vi "Close.vi"(8 "error in":errorcluster, 11 "Current Gradient in":refnum<class "Current Gradient.lvclass">) -> (0 "error out":errorcluster, 3 "Current Gradient out":refnum<class "Current Gradient.lvclass">)   [LabVIEW 2023, in "Current Gradient.lvclass"]
uses:
  Current Gradient.lvclass
  Current Gradient.lvclass/Current Gradient.ctl
  Parents/Gradient/Gradient.lvclass
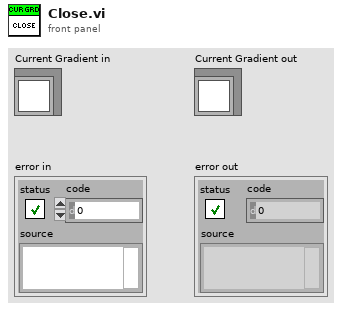
[diagram p1: front panel]
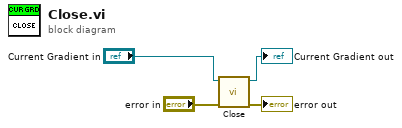
[diagram p0: block diagram]
diagram:
  n1 = call-parent "Close.vi"("error in"="error in", "Gradient in"="Current Gradient in") -> ("error out"=→"error out":errorcluster, "Gradient out"=→"Current Gradient out":refnum<class "Current Gradient.lvclass">)  [unwired: 8 in]
